vi "Set Data.vi"(8 "error in (no error)":errorcluster, 10 "Data":u8[](array[numeric]), 11 "Hex Viewer in":refnum<class "Hex Viewer.lvclass">) -> (0 "error out":errorcluster)   [LabVIEW 2021, in "Hex Viewer.lvclass"]
uses:
  Hex Viewer.lvclass
  Hex Viewer.lvclass/Hex Viewer.ctl
  <userlib>/_OpenG.lib/comparison/comparison.llb/1D U8 Array Changed__ogtk.vi
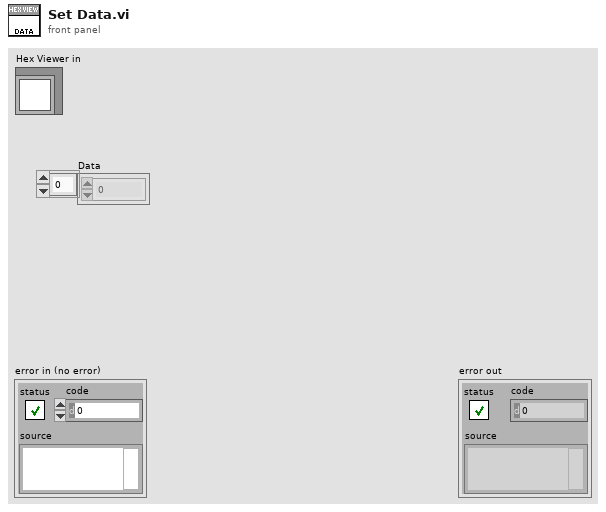
[diagram p1: front panel]
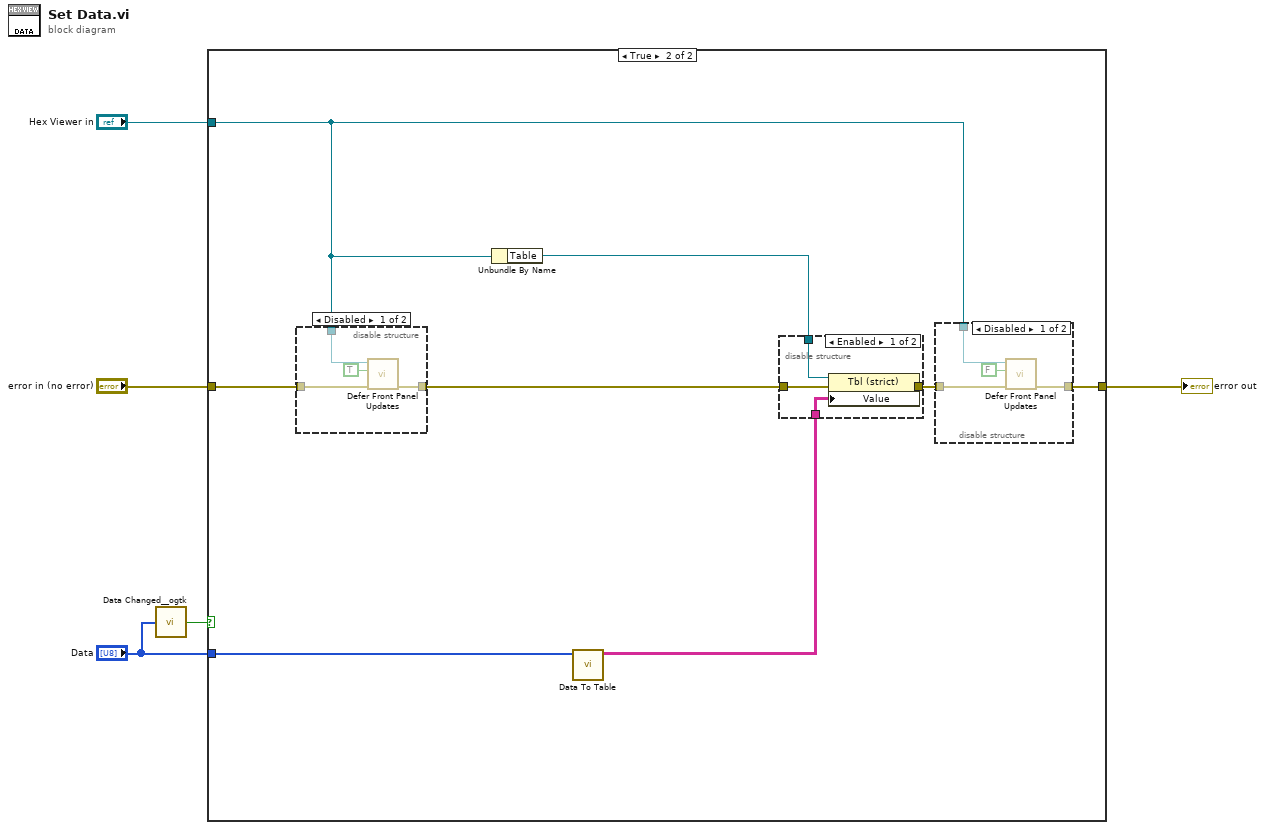
[diagram p0: block diagram]
diagram:
  n1 = call-poly <userlib>:"Data Changed__ogtk.vi"("1D U8 Array"="Data") -> ("Changed"=w1:bool)
  n2 = case shown="True" w1 {
    tunnel: "error in (no error)" -> [w6 w14]
    tunnel: [w6 w9] -> w4
    tunnel: "Hex Viewer in" -> [_ w8]
    tunnel: "Data" -> [_ w7]
    frame False {
    }
    frame True {
      n3 = disable-structure shown="Disabled" {
        disable-tunnel: w14 -> [w26 _]
        disable-tunnel: [w25 _] -> w12
        disable-tunnel: w8 -> [w23 _]
        frame Disabled {
          n4 = call "Defer Front Panel Updates.vi"("error in (no error)"=w26, "Defer"=TRUE, "Hex Viewer in"=w23) -> ("error out"=w25:errorcluster)  [unwired: 8 in]
        }
        frame Enabled {
        }
      }
      n5 = Unbundle By Name(w8) -> ("Table"=w13:refnum<vi>)
      n6 = call "Data To Table.vi"("Data"=w7) -> ("Array"=w11:string[][])  [unwired: 10 in]
      n7 = disable-structure shown="Enabled" {
        disable-tunnel: w13 -> [w18 _]
        disable-tunnel: w12 -> [w17 _]
        disable-tunnel: w11 -> [w16 _]
        disable-tunnel: [w15 _] -> w10
        frame Enabled {
          n8 = property class="Tbl (strict)"(reference=w18, error in=w17, "Value"=w16) -> (error out=w15:errorcluster)  [unwired: 1 out]
        }
        frame Disabled {
        }
      }
      n9 = disable-structure shown="Disabled" {
        disable-tunnel: w10 -> [w21 _]
        disable-tunnel: [w20 _] -> w9
        disable-tunnel: w8 -> [w19 _]
        frame Disabled {
          n10 = call "Defer Front Panel Updates.vi"("error in (no error)"=w21, "Defer"=FALSE, "Hex Viewer in"=w19) -> ("error out"=w20:errorcluster)  [unwired: 8 in]
        }
        frame Enabled {
        }
      }
    }
  }
  "error out" <- w4
